vi "CreateStopEvent.vi"(0 "object in":refnum<class "Application.lvclass">, 5 "error in (no error)":errorcluster) -> (14 "object out":refnum<class "Application.lvclass">, 19 "error out":errorcluster)   [LabVIEW 2019, in "Application.lvclass"]
uses:
  Application.lvclass
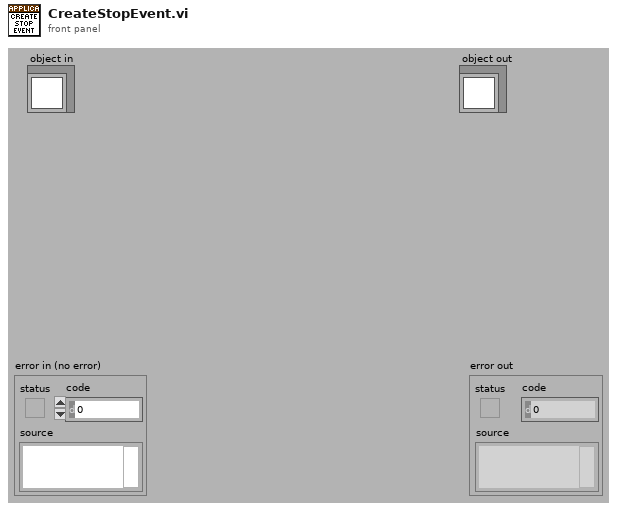
[diagram p1: front panel]
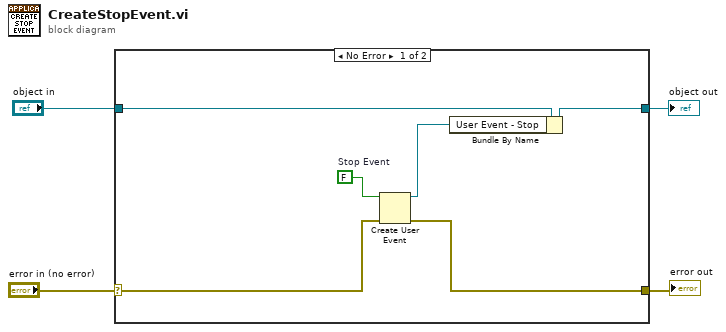
[diagram p0: block diagram]
diagram:
  n1 = case shown="No Error" "error in (no error)" {
    selector: "error in (no error)" -> [w8 w12]
    tunnel: [w7 w12] -> w3
    tunnel: [w6 w11] -> w1
    tunnel: "object in" -> [w10 w11]
    frame No Error {
      w9 = FALSE  # Stop Event
      n2 = Create User Event(user event datatype=w9, error in=w8) -> (user event=w5:refnum<user-event>, error out=w7:errorcluster)
      n3 = Bundle By Name(cluster=w10, "User Event - Stop"=w5) -> (w6:refnum<class "Application.lvclass">)
    }
    frame Error {
    }
  }
  "error out" <- w3
  "object out" <- w1
